vi "Find Modules API Testers.vi"(11 "Module Path":path) -> (0 "error out":errorcluster, 3 "API Testers Paths":path[](array[path]))   [LabVIEW 2016, in "PantherLAB_Scripting.lvlib"]
uses:
  PantherLAB_Scripting.lvlib
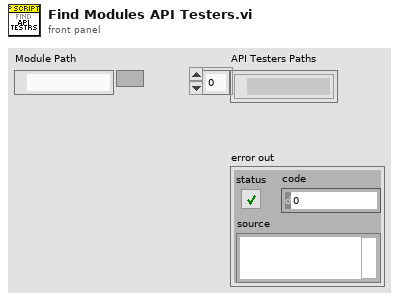
[diagram p1: front panel]
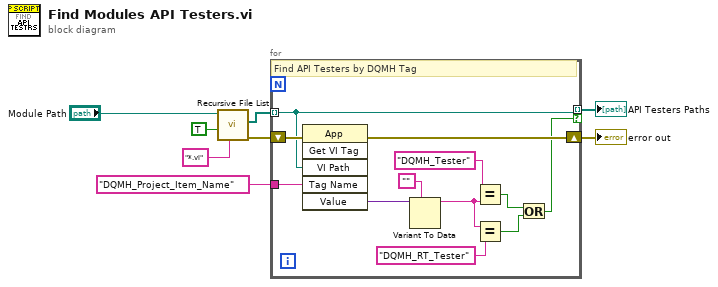
[diagram p0: block diagram]
diagram:
  n1 = call <vilib>:"Recursive File List.vi"("pattern"="*.vi", "Continue Recursing on Error? (F)"=TRUE, "Folder Path"="Module Path") -> ("error out"=w7:errorcluster, "All Files in Dir"=w3:path[])  [unwired: 4 in, 3 out]
  n2 = for {
    tunnel: w3 -> [w10] mode=indexing
    shift-right: [w19] -> w8
    shift-left: w7 -> [w20]
    tunnel: "DQMH_Project_Item_Name" -> [w18]
    tunnel: [w10] -> w5 mode=indexing if=w9
    # "Find API Testers by DQMH Tag"
    n3 = invoke class="App" method="Get VI Tag"(error in=w20, "VI Path"=w10, "Tag Name"=w18) -> (error out=w19:errorcluster, "Value"=w17:variant)  [unwired: 3 in, 4 out]
    n4 = Variant To Data(type="", Variant=w17) -> (data=w13:string)  [unwired: 1 in, 1 out]
    n5 = Equal?(x="DQMH_Tester", y=w13) -> (x = y?=w12:bool)
    n6 = Equal?(x=w13, y="DQMH_RT_Tester" ("x")) -> (x = y?=w11:bool)
    n7 = Or(x=w12, y=w11) -> (x .or. y?=w9:bool)
  }
  "error out" <- w8
  "API Testers Paths" <- w5
